vi "thermo_format_last_values.vi"(1 "force print":bool, 2 "thermo":T1={"type"=enum."COMET Tx5xx (ethernet)", "comment"="", "tag"="", "refresh"=5.0, "IP"="192.168.2.34", "port"=502, "VISA"="", "last readout"=timestamp(0 s since 1904-01-01), "TCP ref"=refnum, "VISA sess"="", "idn"="", "press"=0.0, "RH"=0.0, "temp"=0.0, "pres cor"=[], "RH cor"=[], "temp cor"=[], "try left"=0, "failed"=FALSE, "RTD set"=[], "RTD inv"=[], "range"=0.0, "net mode"=enum."MODBUS", "try fail"=enum."Stop trying - return NaN", "timeout [s]"=0.0, "max retries"=0, "sim t [deg]"=0.0, "status"=0} {"status" items=["ok", "retry", "failed"]; "RTD inv" format="%.1f"; "RTD set" format="%.1f"; "temp cor" format="%.1f"; "RH cor" format="%.1f"; "pres cor" format="%.1f"; "refresh" min=0.1 max=1000.0 format="%.2f"}, 4 "format prefix":string="%.;") -> (5 "temperature":string, 6 "RH":string, 7 "pressure":string)   [LabVIEW 2020]
uses:
  thermo.ctl
  thermo_types.ctl
  Thermometer Fail Action.ctl
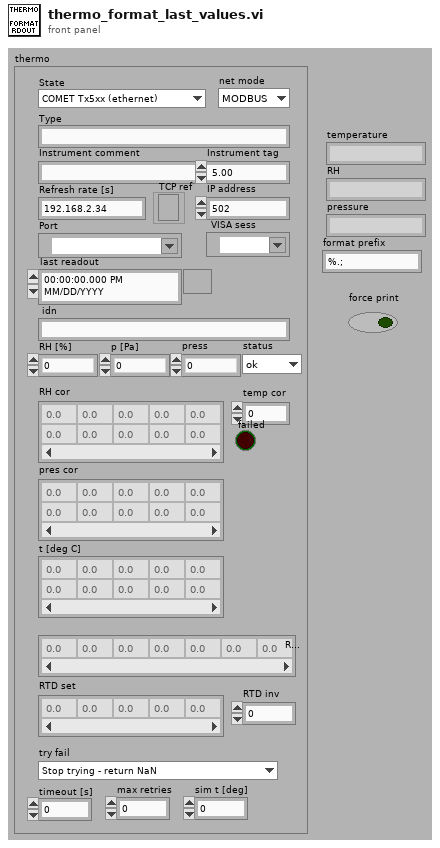
[diagram p1: front panel]
types:
  T1 = typedef "thermo.ctl" = cluster{"type":T2, "comment":string, "tag":string, "refresh":dbl, "IP":string, "port":u16, "VISA":refnum<visa-resource-name>, "last readout":timestamp, "TCP ref":refnum<k5>, "VISA sess":refnum<visa-resource-name>, "idn":string, "press":dbl, "RH":dbl, "temp":dbl, "pres cor":dbl[][], "RH cor":dbl[][], "temp cor":dbl[][], "try left":i32, "failed":bool, "RTD set":dbl[], "RTD inv":dbl[], "range":dbl, "net mode":enum16{"MODBUS", "HTTP"}, "try fail":T3, "timeout [s]":dbl, "max retries":i32, "sim t [deg]":dbl, "status":u16}
  T2 = typedef "thermo_types.ctl" = enum16{"Disabled", "Simulated", "COMET Tx5xx (ethernet)", "Keithley 2002 (GPIB) + RTD", "Agilent 344xx (GPIB) + RTD"}
  T3 = typedef "Thermometer Fail Action.ctl" = enum16{"Stop trying - keep last value", "Stop trying - return NaN", "Generate error - stop sweep"}
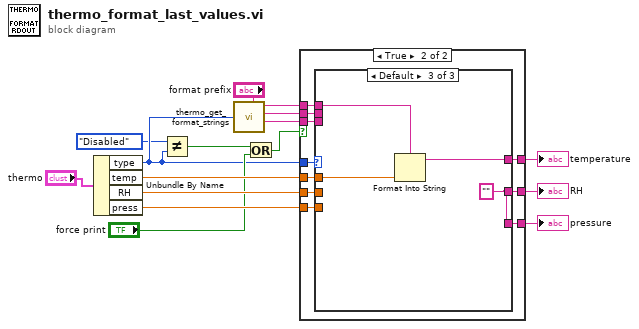
[diagram p0: block diagram]
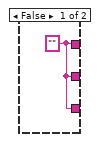
[diagram p2: hidden frame]
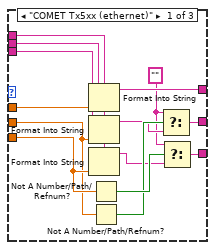
[diagram p3: hidden frame]
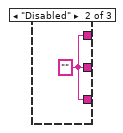
[diagram p4: hidden frame]
diagram:
  n1 = Unbundle By Name("thermo") -> ("type"=w3:T2, "temp"=w15:dbl, "RH"=w14:dbl, "press"=w13:dbl)
  n2 = Not Equal?(x=thermo_types."Disabled", y=w3) -> (x != y?=w2:bool)
  n3 = call "thermo_get_format_strings.vi"("format prefix"="format prefix", "type index"=w3) -> ("pres format"=w4:string, "RH format"=w5:string, "temp format"=w8:string)  [unwired: 1 out]
  n4 = Or(x=w2, y="force print") -> (x .or. y?=w7:bool)
  n5 = case shown="True" w7 {
    tunnel: w3 -> [_ w27]
    tunnel: w15 -> [_ w26]
    tunnel: w8 -> [_ w25]
    tunnel: w14 -> [_ w24]
    tunnel: w13 -> [_ w23]
    tunnel: [w17 w22] -> w12
    tunnel: [w17 w21] -> w11
    tunnel: [w17 w20] -> w10
    tunnel: w5 -> [_ w19]
    tunnel: w4 -> [_ w18]
    frame False {
      w17 = ""
    }
    frame True {
      n6 = case shown="Default" w27 {
        tunnel: w26 -> [w41 _ w46]
        tunnel: w25 -> [w39 _ w45]
        tunnel: w24 -> [w32 _ _]
        tunnel: [w40 w42 w44] -> w22
        tunnel: [w33 w42 w43] -> w21
        tunnel: w23 -> [w37 _ _]
        tunnel: [w38 w42 w43] -> w20
        tunnel: w19 -> [w35 _ _]
        tunnel: w18 -> [w34 _ _]
        frame "COMET Tx5xx (ethernet)" {
          w28 = "" ("f")
          n7 = Format Into String(format string=w39, w41) -> (resulting string=w40:string)  [unwired: 2 in, 1 out]
          n8 = Format Into String(format string=w35, w32) -> (resulting string=w30:string)  [unwired: 2 in, 1 out]
          n9 = Format Into String(format string=w34, w37) -> (resulting string=w29:string)  [unwired: 2 in, 1 out]
          n10 = Not A Number/Path/Refnum?(number/path/refnum=w37) -> (NaN/Path/Refnum?=w36:bool)
          n11 = Not A Number/Path/Refnum?(number/path/refnum=w32) -> (NaN/Path/Refnum?=w31:bool)
          n12 = Select(t=w28, s=w31, f=w30) -> (s? t:f=w33:string)
          n13 = Select(t=w28, s=w36, f=w29) -> (s? t:f=w38:string)
        }
        frame "Disabled" {
          w42 = ""
        }
        frame Default {
          w43 = ""
          n14 = Format Into String(format string=w45, w46) -> (resulting string=w44:string)  [unwired: 2 in, 1 out]
        }
      }
    }
  }
  "temperature" <- w12
  "RH" <- w11
  "pressure" <- w10
